vi "CRYReport Part ObjectSized Event Callback.vi"(4 "TXTextControl":refnum<k7>, 5 "Event Data":cluster{"ObjectId":i16}, 6 "Control Ref":refnum<k7>, 7 "Event Common Data":T1) -> ()   [LabVIEW 2013]
uses:
  CRYReport Global.vi
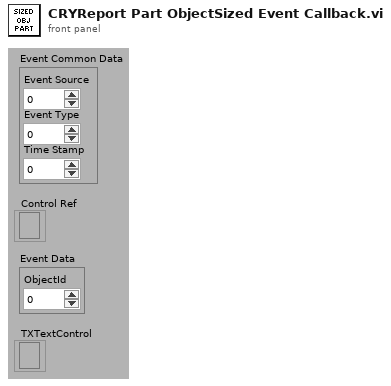
[diagram p1: front panel]
types:
  T1 = cluster{"Event Source":i32, "Event Type":u32, "Time Stamp":u32}
  T2 = cluster{"nID":i16, "sName":string, "pVIRef":refnum<vi>, "pSPRef":refnum<vi>, "sTitle":string, "nIDObject":i16, "nIDV":i16, "nWidth":i16, "nHeight":i16, "bImgChange":bool, "sType":string, "sState":string, "sPosition":string, "sData":string}
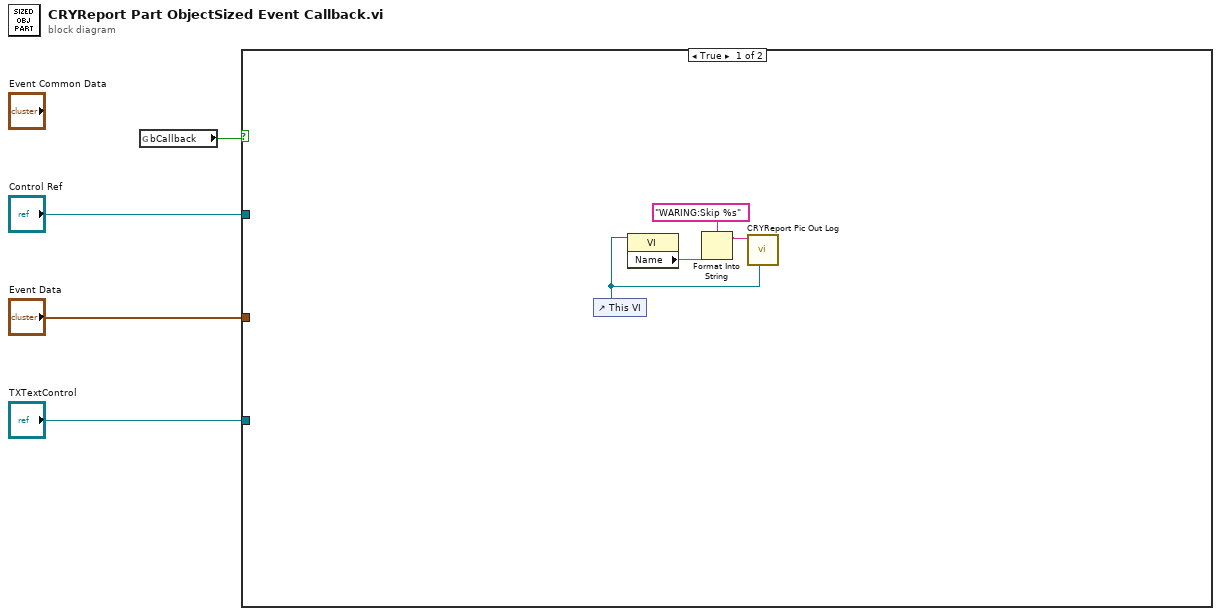
[diagram p0: block diagram]
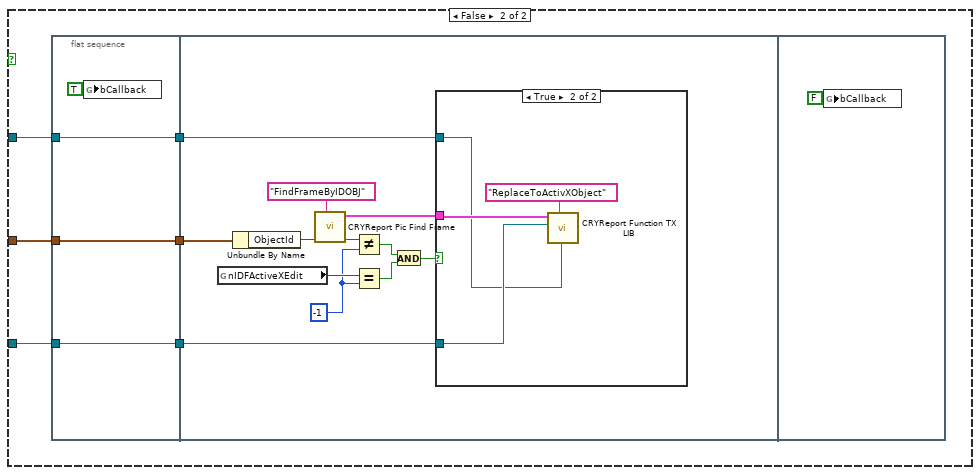
[diagram p2: hidden frame]
diagram:
  n1 = global read "CRYReport Global.vi" "bCallback"() -> (w1:bool)
  n2 = case shown="True" w1 {
    tunnel: "Event Data" -> [_ w11]
    tunnel: "Control Ref" -> [_ w10]
    tunnel: "TXTextControl" -> [_ w9]
    frame True {
      n3 = control-ref of="This VI"() -> (w8:refnum<vi>)
      n4 = property class="VI"(reference=w8) -> ("Name"=w7:string)  [unwired: 1 in, 2 out]
      n5 = Format Into String(format string="WARING:Skip %s" ("string"), w7) -> (resulting string=w5:string)  [unwired: 2 in, 1 out]
      n6 = call "CRYReport Pic Out Log.vi"("vi reference"=w8, "sData"=w5) -> ()  [unwired: 10 in]
    }
    frame False {
      n7 = flat-sequence {
        tunnel: w9 -> [w16]
        tunnel: w10 -> [w17]
        tunnel: w11 -> [w18]
        tunnel: [w18] -> w14
        tunnel: [w17] -> w13
        tunnel: [w16] -> w12
        tunnel: w14 -> [w29]
        tunnel: w13 -> [w20]
        tunnel: w12 -> [w19]
        frame #0 {
          n8 = global write "CRYReport Global.vi" "bCallback"(TRUE ("bCallback")) -> ()
        }
        frame #1 {
          w24 = -1 ("y")
          n9 = global read "CRYReport Global.vi" "nIDFActiveXEdit"() -> (w25:i16)
          n10 = Unbundle By Name(w29) -> ("ObjectId"=w28:i16)
          n11 = call "CRYReport Pic Find Frame.vi"("sAction"="FindFrameByIDOBJ", "nData"=w28) -> ("nData_Out"=w26:i32, "cFrame_Out"=w27:T2)  [unwired: 8 in]
          n12 = Not Equal?(x=w26, y=w24) -> (x != y?=w23:bool)
          n13 = Equal?(x=w25, y=w24) -> (x = y?=w22:bool)
          n14 = And(x=w23, y=w22) -> (x .and. y?=w21:bool)
          n15 = case shown="True" w21 {
            tunnel: w27 -> [_ w33]
            tunnel: w19 -> [_ w32]
            tunnel: w20 -> [_ w31]
            frame False {
            }
            frame True {
              n16 = call "CRYReport Function TX LIB.vi"("Control Ref"=w31, "sAction"="ReplaceToActivXObject", "TXTextControl"=w32, "cFrame"=w33) -> ()  [unwired: 5 in, 3 out]
            }
          }
        }
        frame #2 {
          n17 = global write "CRYReport Global.vi" "bCallback"(FALSE ("bCallback")) -> ()
        }
      }
    }
  }
